vi "RT-Main.vi"() -> ()   [LabVIEW 2020]
doc: "This VI transfers data to and from the FPGA VI to send and receive bytes from an I2C port. <b>Port</b> designates the current port for communication and <b>I2C_Address</b> specifies which slave on the port to communicate with. Place data to write into <b>Write Data</b> and retrieve data from FPGA VI in <b>Read Data</b>."
uses:
  <vilib>/Platform/TimedLoop/XDataNode/timing_clust.ctl
  <vilib>/Platform/TimedLoop/XDataNode/nitl_modes.ctl
  <vilib>/Platform/TimedLoop/XDataNode/wakeup.ctl
  <vilib>/FPGAPlugInAG/myRIO-1900/niLvFpga_Open_myRIO-1900.vi
  <vilib>/Platform/TimedLoop/XDataNode/loadnilvce.vi
  <vilib>/Utility/error.llb/Error Cluster From Error Code.vi
  <vilib>/rvi/errors/niLvFpgaAdjustHostInterfaceError.vi
  <vilib>/FPGAPlugInAG/myRIO-1900/niLvFpga_Close_myRIO-1900.vi
  <vilib>/rvi/interface/nirviOpenFPGA/nirviOpenFPGA.xnode
  Controls/FPGA I2C_FPGA Ref.ctl
  FPGA Bitfiles/I2CCommunication_FPGATarget2_I2CCommunication_VvdNkCkGvgg.lvbitx
  FPGA/FPGA-Main.vi
  <vilib>/platform/TimedLoop/XDataNode/XDataNode.xnode
  <vilib>/rvi/interface/nirviReadWriteControl/nirviReadWriteControl.xnode
  <vilib>/rvi/interface/nirviCloseFPGA/nirviCloseFPGA.xnode
  Library/I2C Host API.lvlib
  NiFpgaLv.dll
  <vilib>/Platform/TimedLoop/XDataNode/XDNodeRunTimeDep.lvlib
panel:
  out "Pressure rounded (mmHg)":dbl format="%.2f"
  out "Temp (F)":sgl
  out "Temp rounded (C)":dbl
  out "Temp (C)":sgl
  out "Scratchpad Data":u8[](array[numeric])
  out "ROM Data":u8[](array[numeric])
  out "Pressure (mmHg)":dbl format="%.2f"
  out "Pressure (PSI)":dbl format="%#.4g"
  out "Pressure (Pa)":dbl format="%#.2g"
  out "Pressure (mbar)":dbl format="%.2f"
  out "Temp (C)":dbl format="%#.2g"
  out "Read Data":u8[](array[numeric])
  out "Error Out":errorcluster
  # "Pressure Sensor"
  # "Status"
  # "Temperature Sensor"
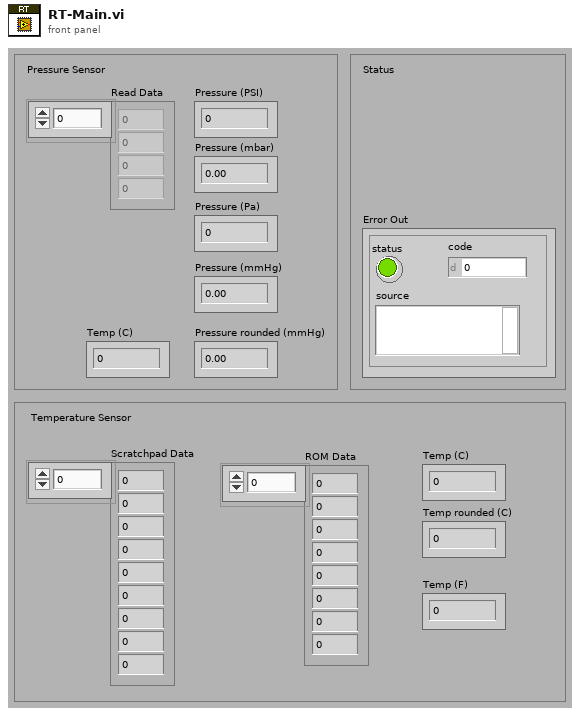
[diagram p1: front panel]
types:
  T1 = typedef "XDNodeRunTimeDep.lvlib/timing_clust.ctl" = cluster{"Expected End [f-1]":u64, "Actual End [f-1]":u64, "Finished Late? [f-1]":bool, "Expected End [i-1]":u64, "Actual End [i-1]":u64, "Finished Late? [i-1]":bool, "Expected Start [i]":u64, "Actual Start [i]":u64, "Expected Start [f]":u64, "Actual Start [f]":u64, "Source Name":string, "Structure Name":string, "Period":i64, "Deadline":i64, "Offset":i64, "Start":i64, "Priority":i32, "Timeout":i32, "Mode":T2, "Wakeup Reason":T3, "Error":errorcluster, "Source Type":string, "Secondary Source Type":string, "Global End Time":u64, "Global Start Time":u64, "Frame Duration":u64, "Iteration Duration":u64, "Assigned CPU":i32, "I/O Scan Engine Mode":u32}
  T2 = typedef "XDNodeRunTimeDep.lvlib/nitl_modes.ctl" = enum32{"No Change", "Process missed periods, maintain original phase", "Discard missed periods, maintain original phase", "Process missed periods, ignore original phase", "Discard missed periods, ignore original phase"}
  T3 = typedef "XDNodeRunTimeDep.lvlib/wakeup.ctl" = enum32{"Normal", "Aborted", "Asynchronous wakeup", "Timing source error", "Timed loop error", "Timeout"}
  T4 = typedef "FPGA I2C_FPGA Ref.ctl" = refnum<k20>
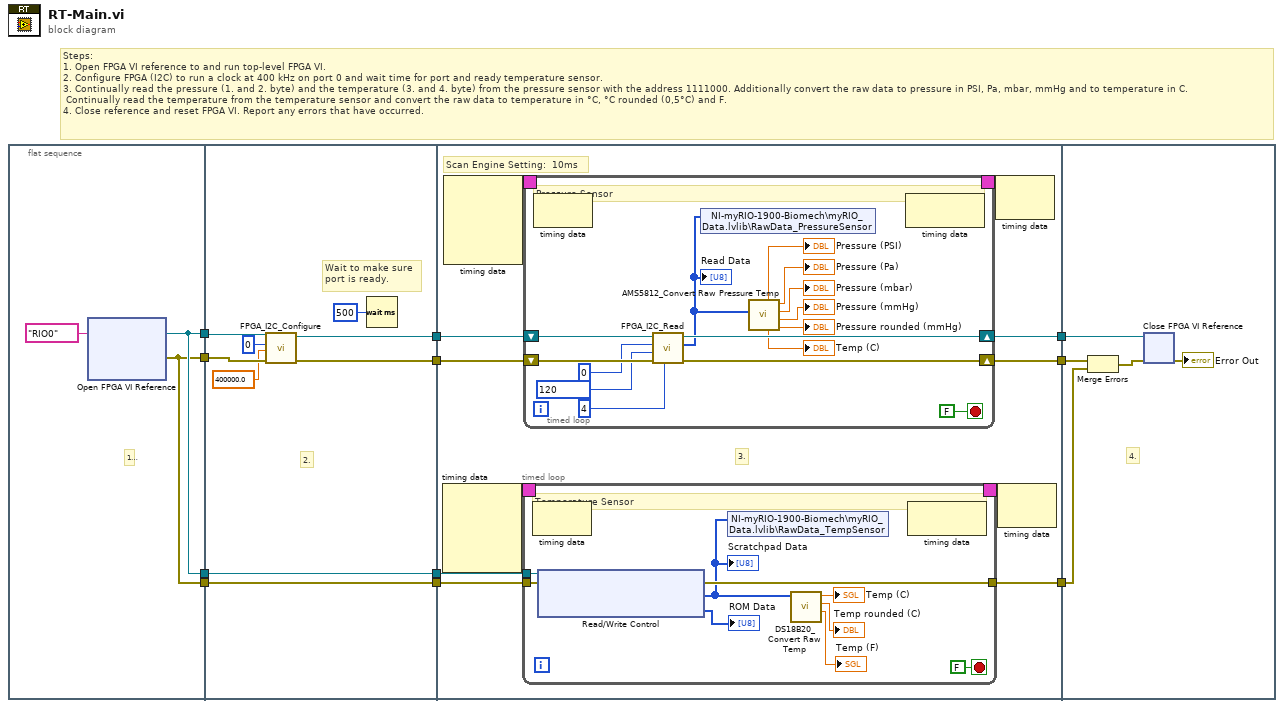
[diagram p0: block diagram]
diagram:
  # "Steps:\n1. Open FPGA VI reference to and run top-level FPGA VI.\n2. Configure FPGA (I2C) to run a clock at 400 kHz on port 0 and wait time for port and ready temperature sensor. \n3. Continually read the pressure (1. and 2. byte) and the temperature (3. and 4. byte) from the pressure sensor with the address 1111000. Additionally convert the raw data to pressure in PSI, Pa, mbar, mmHg and to temperature in C.\n Continually read the temperature from the temperature sensor and convert the raw data to temperature in °C, °C rounded (0,5°C) and F.\n4. Close reference and reset FPGA VI. Report any errors that have occurred."
  n1 = flat-sequence {
    tunnel: [w13] -> w11
    tunnel: [w12] -> w10
    tunnel: [w13] -> w9
    tunnel: [w12] -> w8
    tunnel: w11 -> [w20]
    tunnel: w10 -> [w22]
    tunnel: w9 -> [w17]
    tunnel: w8 -> [w16]
    tunnel: [w22] -> w7
    tunnel: [w17] -> w6
    tunnel: [w21] -> w5
    tunnel: [w16] -> w4
    tunnel: w7 -> [w27]
    tunnel: w6 -> [w30]
    tunnel: w5 -> [w28]
    tunnel: w4 -> [w29]
    tunnel: [w33] -> w3
    tunnel: [w32] -> w2
    tunnel: [w31] -> w1
    tunnel: w3 -> [w67]
    tunnel: w2 -> [w68]
    tunnel: w1 -> [w66]
    frame #0 {
      # "1."
      n2 = xnode "Open FPGA VI Reference"("resource name"=tag "RIO0") -> ("FPGA VI Reference Out"=w13:T4, "error out"=w12:errorcluster)  [unwired: 1 in]
    }
    frame #1 {
      # "Wait to make sure\nport is ready."
      # "2."
      n3 = call "FPGA_I2C_Configure.vi"("error in"=w22, "Clock Rate (Hz)"=400000.0, "Port"=u8 0, "FPGA VI Reference"=w20) -> ("FPGA VI Reference Out"=w21:T4)  [unwired: 7 out]
      n4 = Wait (ms)(milliseconds to wait=u32 500) -> ()  [unwired: 1 out]
    }
    frame #2 {
      # "Scan Engine Setting:  10ms"
      # "3."
      n5 = node-c288() -> (w24:T1)  [unwired: 4 in]
      n6 = node-c288() -> (w26:T1)  [unwired: 4 in]
      n7 = timed-loop {
        tunnel: [w41] -> w33
        tunnel: w30 -> [w36]
        tunnel: w29 -> [w35]
        timing: w24 -> [_]
        timing-out: [_] -> w23
        stop <- FALSE ("stop") stop-if-true
        # "Temperature Sensor"
        n8 = node-c288() -> ()  [unwired: 1 in, 1 out]
        n9 = xnode "Read/Write Control"("FPGA VI Reference In"=w36, "error in"=w35) -> ("error out"=w41:errorcluster, "Scratchpad Data"=w39:u8[], "ROM Data"=→"ROM Data":u8[])  [unwired: 1 out]
        "Scratchpad Data" <- w39
        n10 = shared-variable "NI-myRIO-1900-Biomech\\myRIO_Data.lvlib\\RawData_TempSensor"(w39) -> ()  [unwired: 1 in, 1 out]
        n11 = call "DS18B20_Convert Raw Temp.vi"("Scratchpad Data"=w39) -> ("Temp (F)"=→"Temp (F)":sgl, "Temp rounded (C)"=→"Temp rounded (C)":dbl, "Temp (C)"=→"Temp (C)":sgl)  [unwired: 6 in]
        n12 = node-c288() -> ()  [unwired: 1 in, 1 out]
      }
      n13 = timed-loop {
        shift-right: [w59] -> w32
        shift-left: w27 -> [w60]
        shift-right: [w58] -> w31
        shift-left: w28 -> [w57]
        timing: w26 -> [_]
        timing-out: [_] -> w25
        stop <- FALSE ("Stop") stop-if-true
        # "Pressure Sensor"
        n14 = node-c288() -> ()  [unwired: 1 in, 1 out]
        n15 = call "FPGA_I2C_Read.vi"("Bytes To Read"=u16 4, "error in"=w60, "I2C_Address"=u16 120, "Port"=u8 0, "FPGA VI Reference"=w57) -> ("error out"=w59:errorcluster, "Read Data"=w52:u8[], "FPGA VI Reference Out"=w58:T4)  [unwired: 4 in]
        "Read Data" <- w52
        n16 = shared-variable "NI-myRIO-1900-Biomech\\myRIO_Data.lvlib\\RawData_PressureSensor"(w52) -> ()  [unwired: 1 in, 1 out]
        n17 = call "AMS5812_Convert Raw Pressure Temp.vi"("Read Data"=w52) -> ("Pressure rounded (mmHg)"=→"Pressure rounded (mmHg)":dbl, "Pressure (mmHg)"=→"Pressure (mmHg)":dbl, "Pressure (mbar)"=→"Pressure (mbar)":dbl, "Pressure (Pa)"=→"Pressure (Pa)":dbl, "Temp (C)"=→"Temp (C)":dbl, "Pressure (PSI)"=→"Pressure (PSI)":dbl)  [unwired: 5 in]
        n18 = node-c288() -> ()  [unwired: 1 in, 1 out]
      }
      n19 = node-c288(w25) -> ()  [unwired: 1 out]
      n20 = node-c288(w23) -> ()  [unwired: 1 out]
    }
    frame #3 {
      # "4."
      n21 = Merge Errors(w68, w67) -> (w70:errorcluster)
      n22 = xnode "Close FPGA VI Reference"("FPGA VI Reference In"=w66, "error in"=w70) -> ("error out"=→"Error Out":errorcluster)
    }
  }
